vi "ToFloat.vi"(1 "index":i32, 2 "array":u8[](array[numeric])) -> (0 "sp float":sgl)   [LabVIEW 2010]
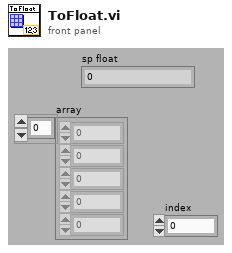
[diagram p1: front panel]
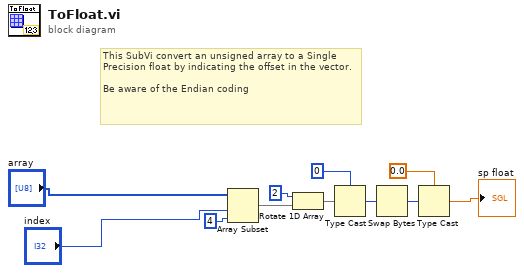
[diagram p0: block diagram]
diagram:
  # "This SubVi convert an unsigned array to a Single Precision float by indicating the offset in the vector.\n\nBe aware of the Endian coding"
  n1 = Array Subset(array="array", index="index", length=4) -> (w7:u8[])
  n2 = Rotate 1D Array(1:w7, 2:2 ("n")) -> (0:w5:u8[])
  n3 = Type Cast(type=u32 0 ("length"), x=w5) -> (*(type *) &x=w3:u32)
  n4 = Swap Bytes(anything=w3) -> (byte swapped=w4:u32)
  n5 = Type Cast(type=sgl 0.0 ("sp float"), x=w4) -> (*(type *) &x=→"sp float":sgl)
